vi "Solve2.vi"(8 "Error In":errorcluster, 11 "object in":refnum<class "2021_17.lvclass">) -> (0 "Error Out":errorcluster, 2 "Result":u64, 3 "object out":refnum<class "2021_17.lvclass">)   [LabVIEW 2020, in "2021_17.lvclass"]
uses:
  2021_17.lvclass
  2021_17.lvclass/2021_17.ctl
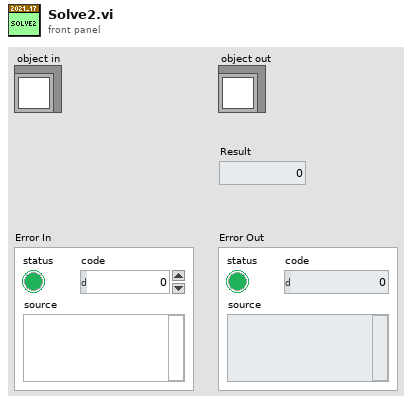
[diagram p1: front panel]
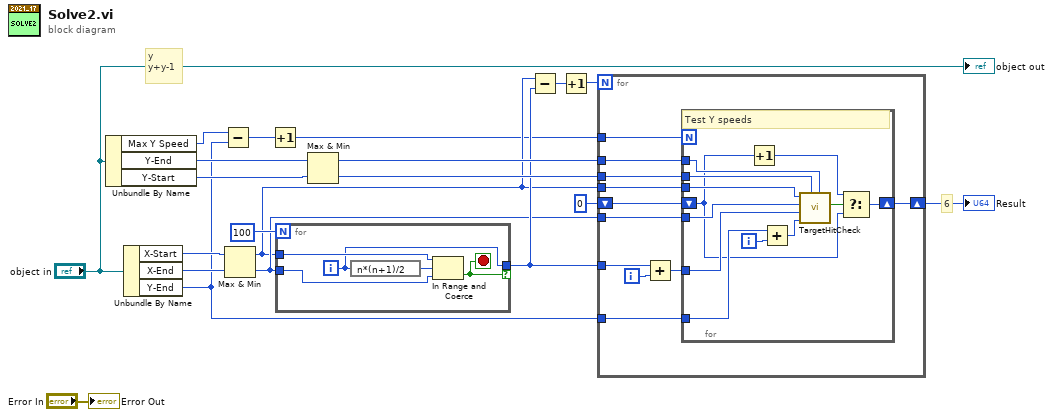
[diagram p0: block diagram]
diagram:
  # "6"
  # "y\ny+y-1"
  n1 = Unbundle By Name("object in") -> ("Max Y Speed"=w6:i32, "Y-End"=w15:i32, "Y-Start"=w14:i32)
  n2 = Unbundle By Name("object in") -> ("X-Start"=w17:i32, "X-End"=w16:i32, "Y-End"=w5:i32)
  n3 = Subtract(x=w6, y=w5) -> (x-y=w4:i32)
  n4 = Max & Min(x=w17, y=w16) -> (max(x,y)=w7:i32, min(x,y)=w8:i32)
  n5 = Increment(x=w4) -> (x+1=w3:i32)
  n6 = for {
    N: 100 -> [_]
    tunnel: w8 -> [w24]
    tunnel: w7 -> [w23]
    tunnel: [w22] -> w11 if=w21
    i -> [w22]
    stop <- w21 stop-if-true
    n7 = expression code="n*(n+1)/2"(w22) -> (w25:i32)
    n8 = In Range and Coerce(upper limit=w23, x=w25, lower limit=w24) -> (In Range?=w21:bool)  [unwired: 1 out]
  }
  n9 = Max & Min(x=w15, y=w14) -> (max(x,y)=w13:i32, min(x,y)=w12:i32)
  n10 = Subtract(x=w7, y=w11) -> (x-y=w10:i32)
  n11 = Increment(x=w10) -> (x+1=w9:i32)
  n12 = for {
    N: w9 -> [_]
    tunnel: w11 -> [w30]
    tunnel: w13 -> [w36]
    tunnel: w12 -> [w35]
    tunnel: w7 -> [w34]
    tunnel: w8 -> [w33]
    tunnel: w5 -> [w29]
    tunnel: w3 -> [w28]
    shift-right: [w26] -> w1
    shift-left: 0 -> [w27]
    i -> [w32]
    n13 = Add(x=w30, y=w32) -> (x+y=w31:i32)
    n14 = for {
      N: w28 -> [_]
      tunnel: w36 -> [w48]
      tunnel: w35 -> [w47]
      tunnel: w31 -> [w44]
      tunnel: w34 -> [w46]
      tunnel: w33 -> [w45]
      tunnel: w29 -> [w43]
      shift-right: [w39] -> w26
      shift-left: w27 -> [w38]
      i -> [w42]
      # "Test Y speeds"
      n15 = Increment(x=w38) -> (x+1=w37:i32)
      n16 = Add(x=w43, y=w42) -> (x+y=w41:i32)
      n17 = call "TargetHitCheck.vi"("Y-Max"=w48, "Y-Min"=w47, "Start Y Speed"=w41, "Start X Speed"=w44, "X-Min"=w45, "X-Max"=w46) -> ("Hit"=w40:bool)  [unwired: 4 in, 1 out]
      n18 = Select(t=w37, s=w40, f=w38) -> (s? t:f=w39:i32)
    }
  }
  "Result" <- w1
  "Error Out" <- "Error In"
  "object out" <- "object in"
